vi "Callback.vi"(10 "Signal Parameter":dbl, 11 "Receiver":refnum<class "LQObject.lvclass">) -> ()   [LabVIEW 2014, in "3c. Connecting a Signal to a LabVIEW Callback.lvlib"]
doc: "The callback VI must have a 4x2x2x4 connector pane with 2 inputs, where the top-left terminal (\"Receiver\") is of LQObject.lvclass type, and the terminal directly below that (\"Signal Parameter\") is of the signal's datatype. However, the \"Signal Parameter\" terminal is omitted for a Void-type callback.\n\nCopyright (c) 2019 Sze Howe Koh.\nThis code is licensed under the MIT license."
uses:
  <vilib>/addons/LQ/LQ Core/LQObject/LQObject.lvclass
  <vilib>/addons/LQ/Qt Widgets/QLCDNumber/QLCDNumber.lvclass
  3c. Connecting a Signal to a LabVIEW Callback.lvlib
panel:
  # "The callback VI must have a 4x2x2x4 connector pane with 2 inputs,\nwhere the top-left terminal (\"Receiver\") is of LQObject.lvclass type,\nand the terminal directly below that (\"Signal Parameter\") is of the\nsignal's datatype. However, the \"Signal Parameter\" terminal is\nomitted for a Void-type callback."
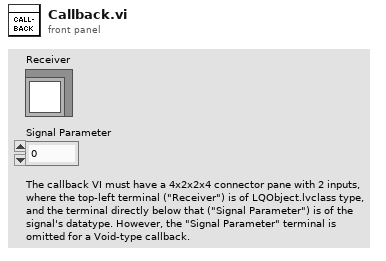
[diagram p1: front panel]
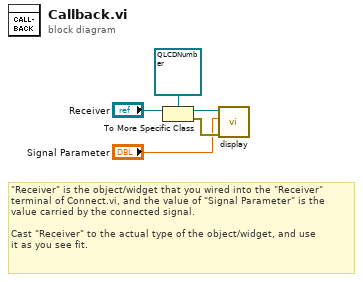
[diagram p0: block diagram]
diagram:
  # "\"Receiver\" is the object/widget that you wired into the \"Receiver\"\nterminal of Connect.vi, and the value of \"Signal Parameter\" is the\nvalue carried by the connected signal.\n\nCast \"Receiver\" to the actual type of the object/widget, and use\nit as you see fit."
  n1 = To More Specific Class(target class=refnum<class "QLCDNumber.lvclass"> refnum ("QLCDNumber"), reference="Receiver") -> (specific class reference=w3:refnum<class "QLCDNumber.lvclass">, error out=w2:errorcluster)  [unwired: 1 in]
  n2 = call <vilib>:"display.vi"("Error In"=w2, "num"="Signal Parameter", "QLCDNumber In"=w3) -> ()  [unwired: 7 in, 2 out]
